vi "q1 equations.vi"() -> ()   [LabVIEW 2018]
panel:
  out "Y":i32
  in  "C":dbl
  in  "B":dbl
  in  "A":sgl
  in  "N":dbl
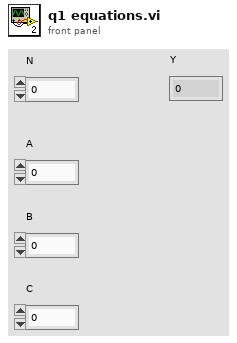
[diagram p1: front panel]
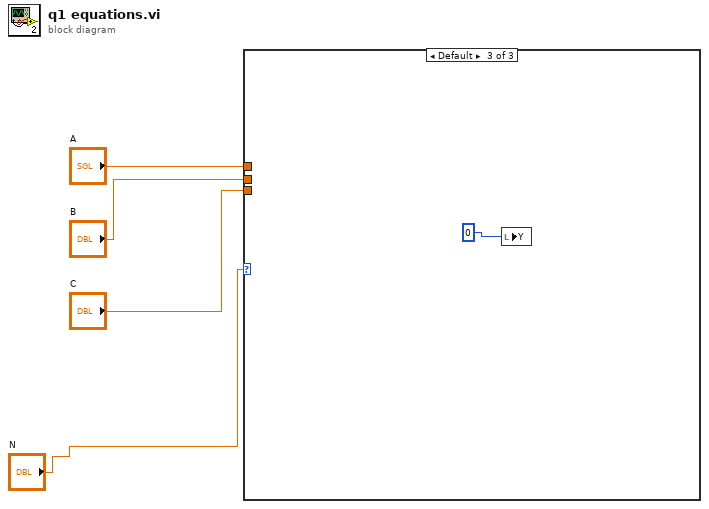
[diagram p0: block diagram]
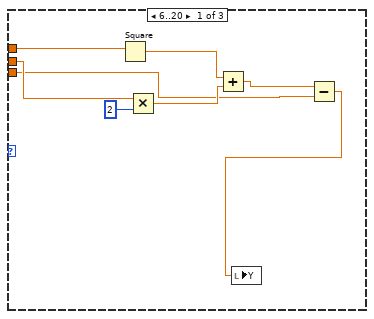
[diagram p2: hidden frame]
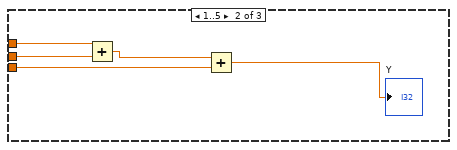
[diagram p3: hidden frame]
diagram:
  n1 = case shown="Default" "N" {
    tunnel: "A" -> [w12 w17 _]
    tunnel: "B" -> [w11 w16 _]
    tunnel: "C" -> [w7 w14 _]
    frame 6..20 {
      n2 = Square(x=w12) -> (x^2=w9:sgl)
      n3 = Multiply(x=w11, y=2) -> (x*y=w8:dbl)
      n4 = Add(x=w9, y=w8) -> (x+y=w6:dbl)
      n5 = Subtract(x=w6, y=w7) -> (x-y=w5:dbl)
      n6 = local write "Y"(w5) -> ()
    }
    frame 1..5 {
      n7 = Add(x=w17, y=w16) -> (x+y=w15:dbl)
      n8 = Add(x=w15, y=w14) -> (x+y=→"Y":dbl)
    }
    frame Default {
      n9 = local write "Y"(0) -> ()
    }
  }
